vi "Tosca-Update CS Mask (new).vi"(0 "Family in":T1) -> (2 "labels":string[][](array[string]), 4 "Family out":T1, 6 "XVar":string, 8 "YVar":string, 10 "Grid":i32[][](array[numeric]))   [LabVIEW 2020]
uses:
  Typedefs/Tosca-Parameter Family.ctl
  Typedefs/Tosca-Parameter Table Element.ctl
  Typedefs/Tosca-Parameter Dimension.ctl
  Typedefs/Tosca-Family Order.ctl
  <vilib>/Analysis/NI_AALPro.lvlib
  <vilib>/Analysis/polynomials.llb/Unique Numbers and Multiplicity (DBL).vi
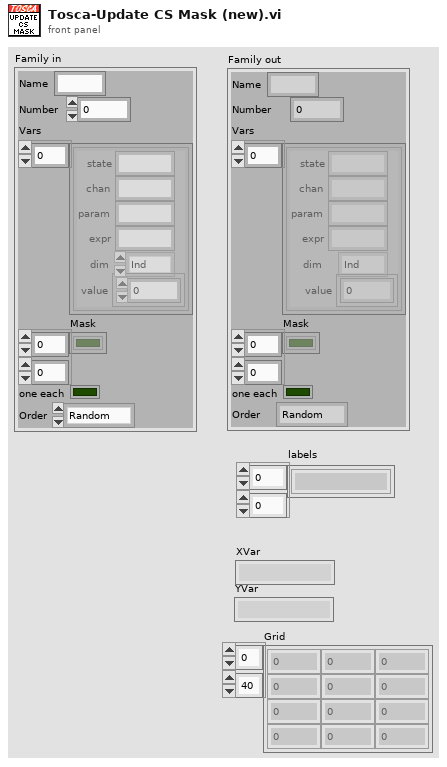
[diagram p1: front panel]
types:
  T1 = typedef "Tosca-Parameter Family.ctl" = cluster{"Name":string, "Number":i32, "Vars":T2[], "Mask":bool[][], "one each":bool, "Order":T4}
  T2 = typedef "Tosca-Parameter Table Element.ctl" = cluster{"state":string, "chan":string, "param":string, "expr":string, "dim":T3, "value":dbl[]}
  T3 = typedef "Tosca-Parameter Dimension.ctl" = enum16{"Ind", "X", "Y"}
  T4 = typedef "Tosca-Family Order.ctl" = enum16{"Random", "Sequential"}
  T5 = cluster{"N":i32, "iOld":i32[], "iNew":i32[], "name":string, "labels":string[]}[]
  T6 = cluster{"N":i32, "iOld":i32[], "iNew":i32[], "name":string, "labels":string[]}
  T7 = cluster{i32, "iA":i32[], "iB":i32[], string, string[]}
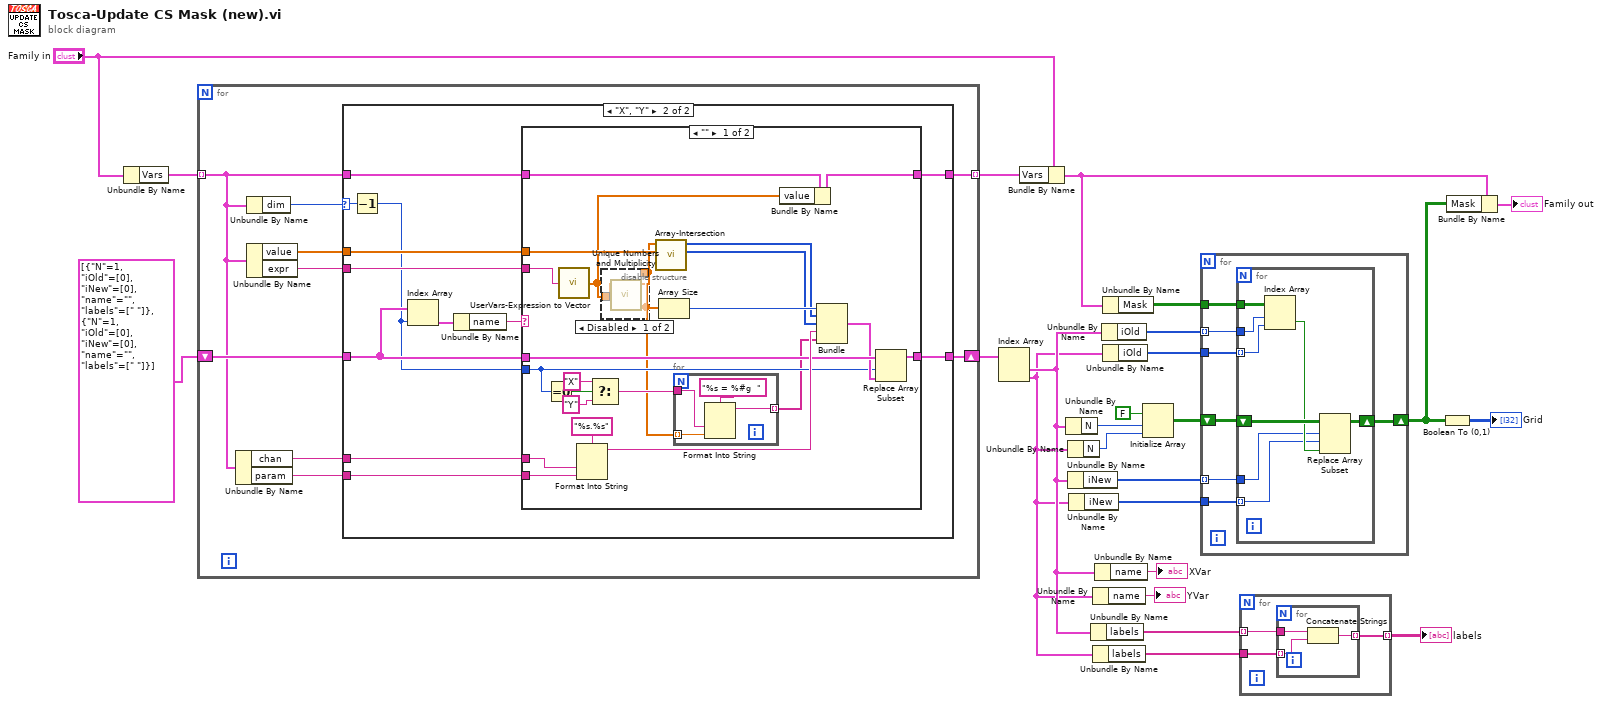
[diagram p0: block diagram]
diagram:
  n1 = Unbundle By Name("Family in") -> ("Vars"=w25:T2[])
  n2 = for {
    tunnel: w25 -> [w28] mode=indexing
    tunnel: [w27] -> w23 mode=indexing
    shift-right: [w26] -> w20
    shift-left: T5 [{"N"=1, "iOld"=[0], "iNew"=[0], "name"="", "labels"=[" "]}, {"N"=1, "iOld"=[0], "iNew"=[0], "name"="", "labels"=[" "]}] -> [w34]
    n3 = Unbundle By Name(w28) -> ("chan"=w33:string, "param"=w32:string)
    n4 = Unbundle By Name(w28) -> ("dim"=w31:T3)
    n5 = Unbundle By Name(w28) -> ("value"=w30:dbl[], "expr"=w29:string)
    n6 = case shown="\"X\", \"Y\"" w31 {
      selector: w31 -> [_ w42]
      tunnel: w34 -> [w35 w39]
      tunnel: w33 -> [_ w48]
      tunnel: w32 -> [_ w47]
      tunnel: w30 -> [_ w46]
      tunnel: w29 -> [_ w45]
      tunnel: w28 -> [w36 w44]
      tunnel: [w36 w43] -> w27
      tunnel: [w35 w37] -> w26
      frame "Ind", Default {
      }
      frame "X", "Y" {
        n7 = Decrement(x=w42) -> (x-1=w38:T3)
        n8 = Index Array(array=w39, index=w38) -> (element=w41:T6)
        n9 = Unbundle By Name(w41) -> ("name"=w40:string)
        n10 = case shown="\"\"" w40 {
          tunnel: w48 -> [w69 _]
          tunnel: w47 -> [w68 _]
          tunnel: w46 -> [w67 _]
          tunnel: w45 -> [w66 _]
          tunnel: w44 -> [w65 w79]
          tunnel: [w64 w79] -> w43
          tunnel: w39 -> [w58 w78]
          tunnel: w38 -> [w55 _]
          tunnel: [w56 w78] -> w37
          frame "" {
            n11 = Equal To 0?(x=w55) -> (x = 0?=w54:bool)
            n12 = call "UserVars-Expression to Vector.vi"("Expr"=w66) -> ("Values"=w63:dbl[])  [unwired: 13 in, 1 out]
            n13 = Format Into String(format string="%s.%s", w69, w68) -> (resulting string=w61:string)  [unwired: 2 in, 1 out]
            n14 = Select(t="X", s=w54, f="Y") -> (s? t:f=w51:string)
            n15 = disable-structure shown="Disabled" {
              disable-tunnel: w63 -> [w72 w73]
              disable-tunnel: [w71 w73] -> w50
              frame Disabled {
                n16 = call-poly <vilib>:"Unique Numbers and Multiplicity.vi"("Numbers"=w72) -> ("Unique Numbers"=w71:dbl[])  [unwired: 8 in, 2 out]
              }
              frame Enabled {
              }
            }
            n17 = call "Array-Intersection.vi"("B"=w67, "A"=w50) -> ("iB"=w59:i32[], "iA"=w60:i32[])  [unwired: 7 in, 1 out]
            n18 = Array Size(array=w50) -> (size(s)=w62:i32)
            n19 = for {
              tunnel: w51 -> [w76]
              tunnel: w50 -> [w75] mode=indexing
              tunnel: [w74] -> w49 mode=indexing
              n20 = Format Into String(format string="%s = %#g  ", w76, w75) -> (resulting string=w74:string)  [unwired: 2 in, 1 out]
            }
            n21 = Bundle By Name(cluster=w65, "value"=w63) -> (w64:T2)
            n22 = Bundle(w62, "iA"=w60, "iB"=w59, w61, w49) -> (w57:T7)  [unwired: 1 in]
            n23 = Replace Array Subset(array=w58, new element=w57, index=w55) -> (w56:T5)
          }
          frame "1", Default {
          }
        }
      }
    }
  }
  n24 = Index Array(array=w20) -> (element #1=w5:T6, element #2=w4:T6)  [unwired: 2 in]
  n25 = Bundle By Name(cluster="Family in", "Vars"=w23) -> (w22:T1)
  n26 = Unbundle By Name(w5) -> ("N"=w18:i32)
  n27 = Unbundle By Name(w4) -> ("N"=w15:i32)
  n28 = Unbundle By Name(w5) -> ("iNew"=w11:i32[])
  n29 = Unbundle By Name(w4) -> ("iNew"=w10:i32[])
  n30 = Unbundle By Name(w5) -> ("labels"=w3:string[])
  n31 = Unbundle By Name(w4) -> ("name"=→"YVar":string)
  n32 = Unbundle By Name(w4) -> ("labels"=w2:string[])
  n33 = Unbundle By Name(w5) -> ("name"=→"XVar":string)
  n34 = Unbundle By Name(w5) -> ("iOld"=w12:i32[])
  n35 = Unbundle By Name(w22) -> ("Mask"=w13:bool[][])
  n36 = Unbundle By Name(w4) -> ("iOld"=w9:i32[])
  n37 = Initialize Array(FALSE, w18, w15) -> (w14:bool[][])
  n38 = for {
    shift-right: [w80] -> w7
    shift-left: w14 -> [w81]
    tunnel: w13 -> [w82]
    tunnel: w12 -> [w84] mode=indexing
    tunnel: w11 -> [w85] mode=indexing
    tunnel: w10 -> [w86]
    tunnel: w9 -> [w83]
    n39 = for {
      tunnel: w86 -> [w87] mode=indexing
      tunnel: w85 -> [w88]
      tunnel: w84 -> [w93]
      tunnel: w83 -> [w92] mode=indexing
      tunnel: w82 -> [w94]
      shift-right: [w90] -> w80
      shift-left: w81 -> [w91]
      n40 = Index Array(array=w94, index (row)=w93, index (col)=w92) -> (element=w89:bool)
      n41 = Replace Array Subset(array=w91, new element=w89, index (row)=w88, index (col)=w87) -> (w90:bool[][])
    }
  }
  n42 = for {
    tunnel: w3 -> [w97] mode=indexing
    tunnel: w2 -> [w96]
    tunnel: [w95] -> w1 mode=indexing
    n43 = for {
      tunnel: w97 -> [w100]
      tunnel: w96 -> [w99] mode=indexing
      tunnel: [w98] -> w95 mode=indexing
      n44 = Concatenate Strings(w100, w99) -> (w98:string)
    }
  }
  "labels" <- w1
  n45 = Boolean To (0,1)(Boolean=w7) -> (0, 1=→"Grid":i16[][])
  n46 = Bundle By Name(cluster=w22, "Mask"=w7) -> (→"Family out":T1)
